vi "MulticolumnView.vi"(6 "CountClear":bool, 8 "VCI_CAN_OBJ_N":T1(array[cluster]), 9 "Num":u32, 10 "MCListbox引用句柄":refnum<vi>, 11 "Tx_Or_Rx":bool) -> (3 "MCListbox输出":refnum<vi>)   [LabVIEW 2013]
uses:
  GlobalVariable.vi
panel:
  out "TRCount":u32
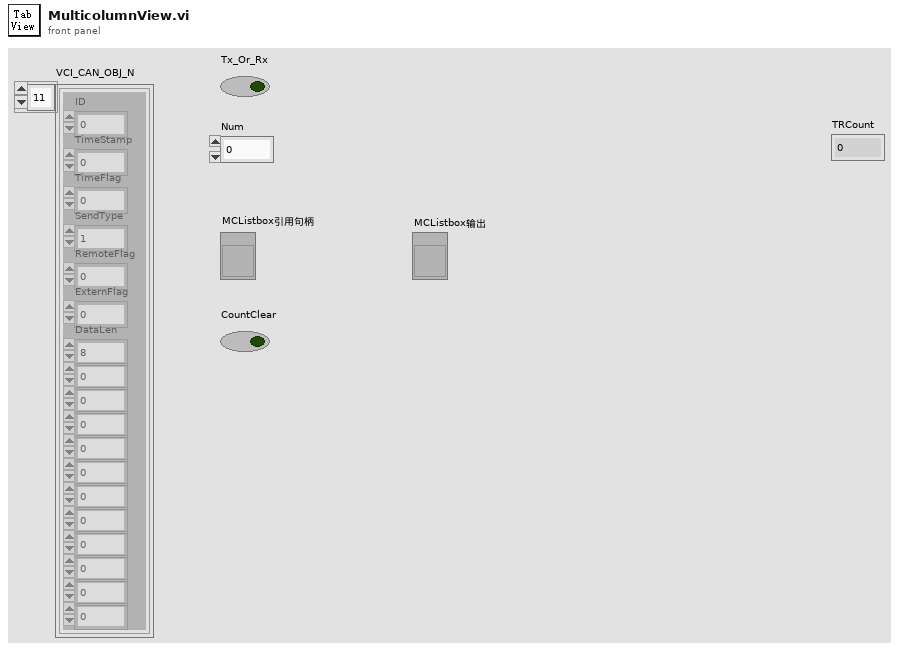
[diagram p1: front panel]
types:
  T1 = cluster{"ID":u32, "TimeStamp":u32, "TimeFlag":u8, "SendType":u8, "RemoteFlag":u8, "ExternFlag":u8, "DataLen":u8, u8, u8, u8, u8, u8, u8, u8, u8, u8, u8, u8}[]
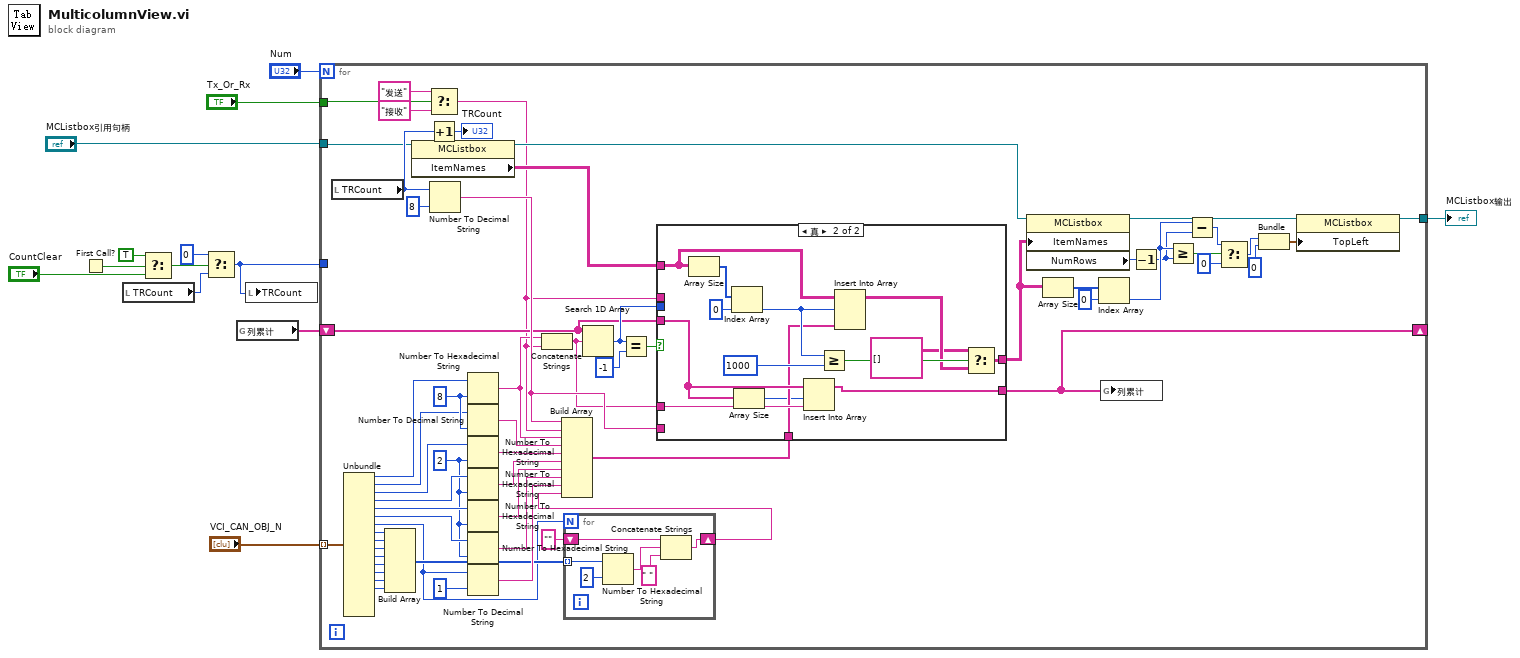
[diagram p0: block diagram]
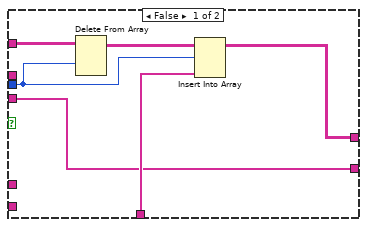
[diagram p2: hidden frame]
diagram:
  n1 = First Call?() -> (First Call?: T/F=w2:bool)
  n2 = local read "TRCount"() -> (w8:u32)
  n3 = Select(t=TRUE, s=w2, f="CountClear") -> (s? t:f=w5:bool)
  n4 = Select(t=0, s=w5, f=w8) -> (s? t:f=w9:u32)
  n5 = global read "GlobalVariable.vi" "列累计"() -> (w3:string[])
  n6 = local write "TRCount"(w9) -> ()
  n7 = for {
    N: "Num" -> [_]
    tunnel: "VCI_CAN_OBJ_N" -> [w43] mode=indexing
    tunnel: "Tx_Or_Rx" -> [w40]
    tunnel: "MCListbox引用句柄" -> [w38]
    tunnel: w9 -> [_]
    tunnel: [w23] -> w7
    shift-right: [w14] -> _
    shift-left: w3 -> [w18]
    w52 = 2
    w73 = 8
    n8 = local read "TRCount"() -> (w44:u32)
    n9 = Unbundle(w43) -> ("ID"=w74:u32, "TimeStamp"=w72:u32, "TimeFlag"=w53:u8, "SendType"=w70:u8, "RemoteFlag"=w71:u8, "ExternFlag"=w69:u8, "DataLen"=w45:u8, w62:u8, w61:u8, w60:u8, w59:u8, w58:u8, w57:u8, w55:u8, w56:u8)  [unwired: 3 out]
    n10 = Build Array(w62, w61, w60, w59, w58, w57, w55, w56) -> (w46:u8[])
    n11 = property class="MCListbox"(reference=w38) -> (reference out=w37:refnum<vi>, "ItemNames"=w39:string[][])  [unwired: 1 in, 1 out]
    n12 = Select(t="发送", s=w40, f="接收") -> (s? t:f=w16:string)
    n13 = Increment(x=w44) -> (x+1=→"TRCount":u32)
    n14 = Number To Decimal String(number=w44, width (-)=i16 8) -> (decimal integer string=w19:string)
    n15 = Number To Hexadecimal String(1:w73, 2:w74) -> (0:w17:string)
    n16 = Number To Decimal String(number=w72, width (-)=w73) -> (decimal integer string=w68:string)
    n17 = Number To Hexadecimal String(1:w52, 2:w53) -> (0:w54:string)
    n18 = Number To Hexadecimal String(1:w52, 2:w70) -> (0:w67:string)
    n19 = Number To Hexadecimal String(1:w52, 2:w71) -> (0:w66:string)
    n20 = Number To Hexadecimal String(1:w52, 2:w69) -> (0:w65:string)
    n21 = Number To Decimal String(number=w45, width (-)=1) -> (decimal integer string=w63:string)
    n22 = Concatenate Strings(w17, w16) -> (w15:string)
    n23 = for {
      N: w45 -> [_]
      shift-right: [w97] -> w48
      shift-left: "" -> [w95]
      tunnel: w46 -> [w96] mode=indexing
      n24 = Number To Hexadecimal String(1:i16 2 ("width (-)"), 2:w96) -> (0:w99:string)
      n25 = Concatenate Strings(w95, w99, " " ("string")) -> (w97:string)
    }
    n26 = Build Array(w19, w16, w17, w68, w54, w67, w66, w65, w63, w48) -> (w51:string[])
    n27 = Search 1D Array(1D array=w18, element=w15) -> (index of element=w20:i32)  [unwired: 1 in]
    n28 = Equal?(x=w20, y=-1) -> (x = y?=w22:bool)
    n29 = case shown="真" w22 {
      tunnel: w51 -> [w80 w83]
      tunnel: w39 -> [w78 w87]
      tunnel: [w79 w86] -> w31
      tunnel: w18 -> [w75 w84]
      tunnel: w15 -> [_ w85]
      tunnel: w20 -> [w77 _]
      tunnel: w16 -> [_ _]
      tunnel: w19 -> [_ _]
      tunnel: [w75 w81] -> w14
      frame False {
        n30 = Delete From Array(array=w78, index (row)=w77) -> (array with subset deleted=w76:string[][])  [unwired: 2 in, 1 out]
        n31 = Insert Into Array(array=w76, index (row)=w77, new element=w80) -> (w79:string[][])  [unwired: 1 in]
      }
      frame True {
        n32 = Array Size(array=w87) -> (size(s)=w93:i32[])
        n33 = Index Array(array=w93, index=0) -> (element=w88:i32)
        n34 = Array Size(array=w84) -> (size(s)=w82:i32)
        n35 = Insert Into Array(array=w84, index=w82, new element=w85) -> (w81:string[])
        n36 = Greater Or Equal?(x=w88, y=1000) -> (x >= y?=w92:bool)
        n37 = Insert Into Array(array=w87, index (row)=w88, new element=w83) -> (w91:string[][])  [unwired: 1 in]
        n38 = Select(t=string[][] [], s=w92, f=w91) -> (s? t:f=w86:string[][])
      }
    }
    n39 = property class="MCListbox"(reference=w37, "ItemNames"=w31) -> (reference out=w35:refnum<vi>, "NumRows"=w28:u32)  [unwired: 1 in, 1 out]
    n40 = Array Size(array=w31) -> (size(s)=w30:i32[])
    n41 = Index Array(array=w30, index=0) -> (element=w27:i32)
    n42 = global write "GlobalVariable.vi" "列累计"(w14) -> ()
    n43 = Decrement(x=w28) -> (x-1=w24:u32)
    n44 = Greater Or Equal?(x=w27, y=w24) -> (x >= y?=w36:bool)
    n45 = Subtract(x=w27, y=w24) -> (x-y=w33:u32)
    n46 = Select(t=w33, s=w36, f=u32 0) -> (s? t:f=w25:u32)
    n47 = Bundle(w25, 0) -> (w34:cluster{u32, i32})  [unwired: 1 in]
    n48 = property class="MCListbox"(reference=w35, "TopLeft"=w34) -> (reference out=w23:refnum<vi>)  [unwired: 1 in, 1 out]
  }
  "MCListbox输出" <- w7
